vi "ErrorHandling_Main.vi"(8 "error in (no error)":errorcluster) -> (0 "error out":errorcluster)   [LabVIEW 2013]
doc: "This is Top Level VI for Error Handling Module. You can communicate with this module using its API. Communication is made based on queue. This module has not User Interface so I chase State Machine architecture."
uses:
  General/Controls/#TD_General_CommunicationQueueStates_Enum.ctl
  Private controls/#TD_ErrorHandling_InnerData_Cluster.ctl
  Private controls/#TD_ErrorHandling_ModuleStates_Enum.ctl
  Private controls/#TD_ErrorHandling_ModuleData_Cluster.ctl
  General/Controls/#TD_General_FromWho_Enum.ctl
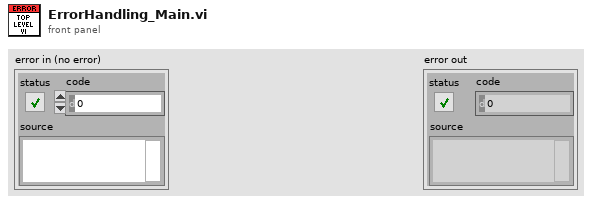
[diagram p1: front panel]
types:
  T1 = typedef "#TD_General_CommunicationQueueStates_Enum.ctl" = enum16{"ERROR_Default", "Obtain", "GetRef", "Enqueue", "EnqueueAtOpp", "GetStatus", "Release"}
  T2 = typedef "#TD_General_FromWho_Enum.ctl" = enum16{"ERROR_Default", "UserConsole", "DisplayConsole", "SensorInterface", "Controller", "Database", "Timing", "ErrorHandling"}
  T3 = typedef "#TD_ErrorHandling_ModuleStates_Enum.ctl" = enum16{"ERROR_Default", "Init", "Close", "ErrorHandling"}
  T4 = typedef "#TD_ErrorHandling_ModuleData_Cluster.ctl" = cluster{"Action":T3, "Data":variant}
  T5 = typedef "#TD_General_IntermoduleData_Cluster.ctl" = cluster{"Sender":T2, "ModuleData":variant}
  T6 = typedef "#TD_ErrorHandling_InnerData_Cluster.ctl" = cluster{"Sth":bool}
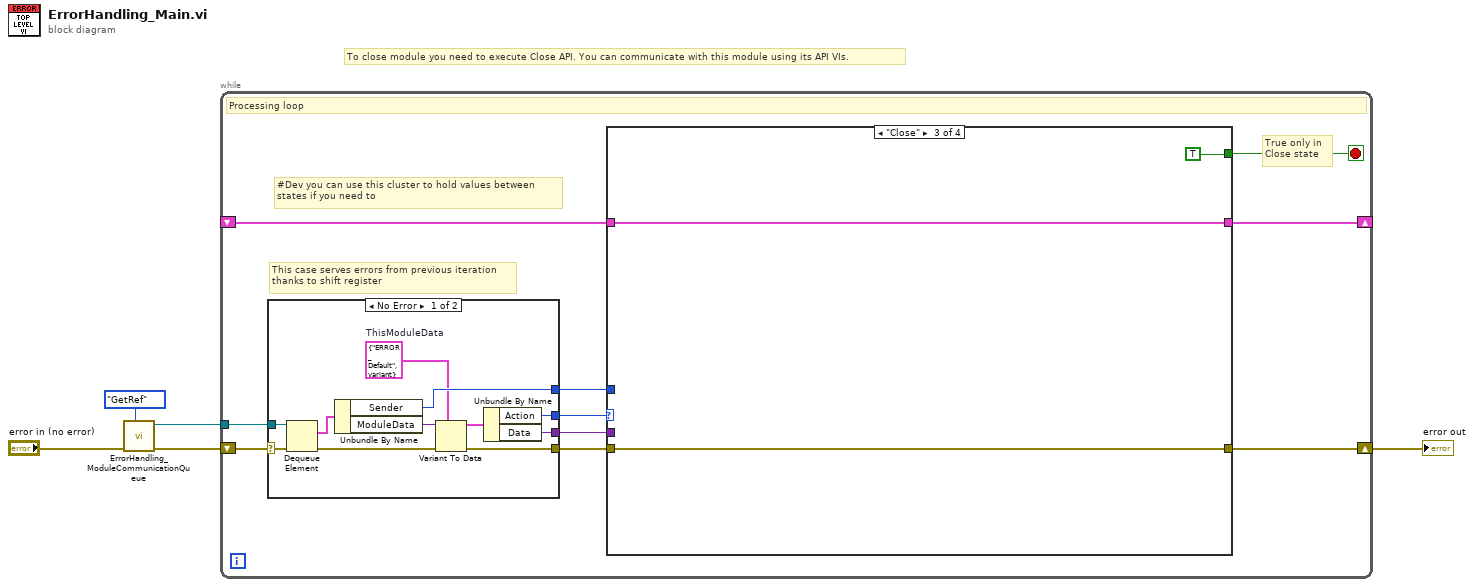
[diagram p0: block diagram]
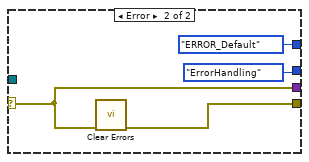
[diagram p2: hidden frame]
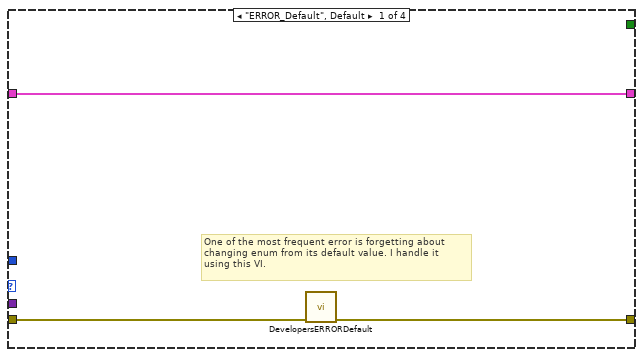
[diagram p3: hidden frame]
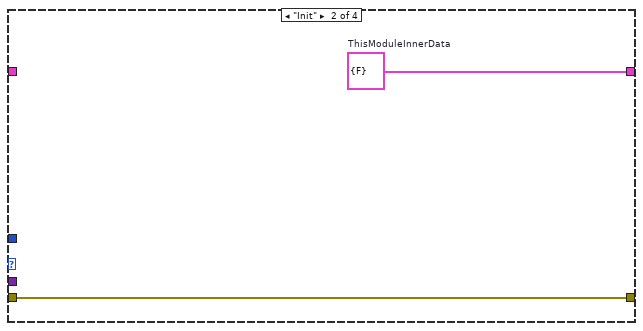
[diagram p4: hidden frame]
diagram:
  # "To close module you need to execute Close API. You can communicate with this module using its API VIs."
  n1 = call "ErrorHandling_ModuleCommunicationQueue.vi"("Action"=#TD_General_CommunicationQueueStates_Enum."GetRef", "error in (no error)"="error in (no error)") -> ("error out"=w2:errorcluster, "Ref out"=w3:refnum<queue>)  [unwired: 7 in, 1 out]
  n2 = while {
    tunnel: w3 -> [w14]
    shift-right: [w7] -> w1
    shift-left: w2 -> [w15]
    shift-right: [w13] -> _
    shift-left: _ -> [w12]
    stop <- w6 stop-if-true
    # "True only in \nClose state"
    # "#Dev you can use this cluster to hold values between \nstates if you need to"
    # "This case serves errors from previous iteration \nthanks to shift register"
    # "Processing loop"
    n3 = case shown="No Error" w15 {
      selector: w15 -> [w26 w30]
      tunnel: w14 -> [w25 _]
      tunnel: [w21 #TD_General_FromWho_Enum."ERROR_Default" ("Sender")] -> w11
      tunnel: [w18 #TD_ErrorHandling_ModuleStates_Enum."ErrorHandling" ("Action")] -> w10
      tunnel: [w17 w30] -> w9
      tunnel: [w16 w29] -> w8
      frame No Error {
        w20 = T4 {"Action"=enum."ERROR_Default", "Data"=variant}  # ThisModuleData
        n4 = Dequeue Element(queue=w25, error in (no error)=w26) -> (element=w24:T5, error out=w22:errorcluster)  [unwired: 1 in, 2 out]
        n5 = Unbundle By Name(w24) -> ("Sender"=w21:T2, "ModuleData"=w23:variant)
        n6 = Variant To Data(error in=w22, type=w20, Variant=w23) -> (data=w19:T4, error out=w16:errorcluster)
        n7 = Unbundle By Name(w19) -> ("Action"=w18:T3, "Data"=w17:variant)
      }
      frame Error {
        n8 = call <vilib>:"Clear Errors.vi"("error in (no error)"=w30) -> ("error out"=w29:errorcluster)  [unwired: 5 in, 1 out]
      }
    }
    n9 = case shown="\"Close\"" w10 {
      tunnel: [w33 w35 w37 w40] -> w13
      tunnel: w12 -> [w33 _ w37 w40]
      tunnel: w11 -> [_ _ _ _]
      tunnel: w9 -> [_ _ _ _]
      tunnel: w8 -> [w32 w34 w36 w39]
      tunnel: [w31 w34 w36 w39] -> w7
      tunnel: [_ _ TRUE _] -> w6
      frame "ERROR_Default", Default {
        # "One of the most frequent error is forgetting about \nchanging enum from its default value. I handle it \nusing this VI."
        n10 = call "DevelopersERRORDefault.vi"("error in (no error)"=w32) -> ("error out"=w31:errorcluster)  [unwired: 10 in]
      }
      frame "Init" {
        w35 = T6 {"Sth"=FALSE}  # ThisModuleInnerData
      }
      frame "Close" {
      }
      frame "ErrorHandling" {
        # "#Dev take some actions to handle the error \nand inform central Error Handling Module \nabout this error using Error Handling Module \nAPI"
      }
    }
  }
  "error out" <- w1
